vi "IDN.vi"(8 "error in (no error)":errorcluster, 11 "Instrument in":refnum<class "Instrument.lvclass">) -> (0 "error out":errorcluster, 2 "IDN":T1, 3 "Instrument in":refnum<class "Instrument.lvclass">)   [LabVIEW 2019, in "Instrument.lvlib" / "Instrument.lvclass"]
doc: "Send \"HELP\" command to get API supported by remote Instrument."
uses:
  Instrument.lvclass
  Typedefs/Instrument.IDN--cluster.ctl
  Typedefs/Instrument.Commands--Enum.ctl
  df6d36b1-df84-4a1a-80e3-72715317c370.vi
  df6d36b1-df84-4a1a-80e3-72715317c370.vi/f656c00c-c0f2-412a-af07-0e63097bf420.vi
  df6d36b1-df84-4a1a-80e3-72715317c370.vi/dea3fd55-9b31-4ef8-901c-88ea68cff87a.vi
  <vilib>/Utility/Data Type/Get Type Information.vi
  <vilib>/JDP Science/JSONtext/JSON text to Variant.vi
  <vilib>/JDP Science/JSONtext/LVClass Serializer/JSONtext LVClass Serializer.lvclass
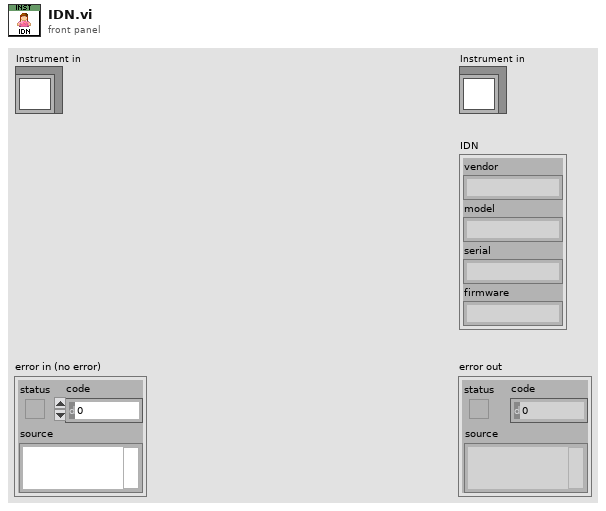
[diagram p1: front panel]
types:
  T1 = typedef "Instrument.lvlib/Instrument.lvclass/Instrument.IDN--cluster.ctl" = cluster{"vendor":string, "model":string, "serial":string, "firmware":string}
  T2 = typedef "Instrument.lvlib/Instrument.lvclass/Instrument.Commands--Enum.ctl" = enum16{"ACK", "HELP", "IDN", "getAll", "getAllData"}
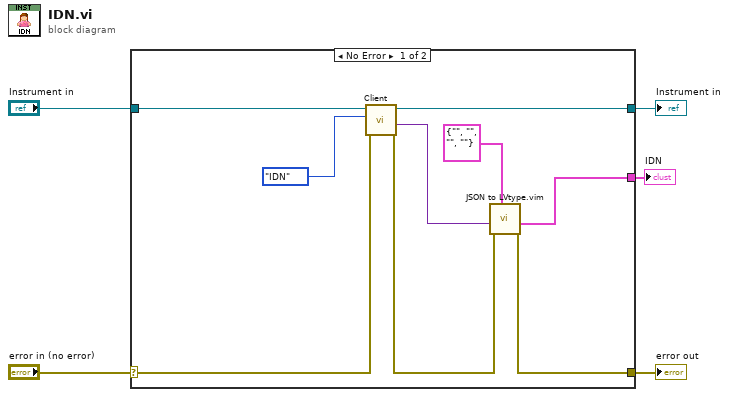
[diagram p0: block diagram]
diagram:
  n1 = case shown="No Error" "error in (no error)" {
    selector: "error in (no error)" -> [w12 w16]
    tunnel: [w9 w16] -> w4
    tunnel: [w14 w15] -> w2
    tunnel: "Instrument in" -> [w13 w15]
    tunnel: [w7 _] -> w1
    frame No Error {
      n2 = call-dynamic "Client.vi"("error in (no error)"=w12, "Command in"=Instrument.Commands--Enum."IDN" ("Commands"), "Instrument in"=w13) -> ("error out"=w10:errorcluster, "Data out"=w8:variant, "Instrument out"=w14:refnum<class "Instrument.lvclass">)  [unwired: 5 in, 1 out]
      n3 = call "JSON to LVtype.vim"("type"=T1 {"vendor"="", "model"="", "serial"="", "firmware"=""} ("IDN"), "error in (no error)"=w10, "JSON Data in"=w8) -> ("error out"=w9:errorcluster, "Data out"=w7:T1)  [unwired: 7 in]
    }
    frame Error {
    }
  }
  "error out" <- w4
  "Instrument in" <- w2
  "IDN" <- w1
